vi "set_controls_enabled_state.vi"(8 "error in (no error)":errorcluster, 9 "status":T1(ring), 10 "control references":refnum<vi>[](array[refnum]), 11 "GenericPlugin in":refnum<class "GenericComponent.lvclass">) -> (0 "error out":errorcluster, 3 "GenericPlugin out":refnum<class "GenericComponent.lvclass">)   [LabVIEW 2010, in "GenericComponent.lvclass"]
uses:
  GenericComponent.lvclass
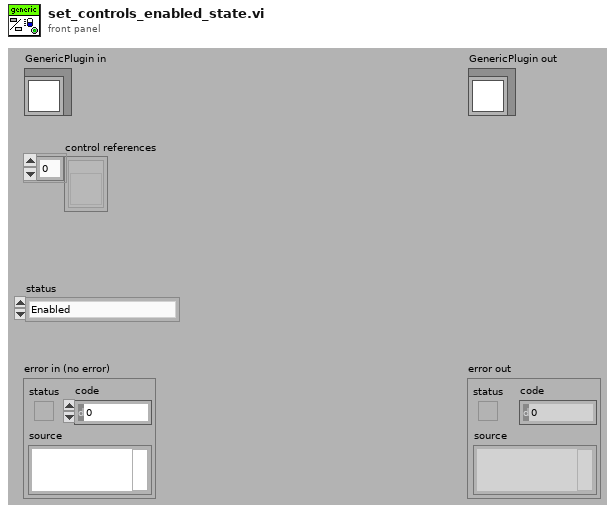
[diagram p1: front panel]
types:
  T1 = enum8{"Enabled", "Disabled", "Disabled and Grayed Out"}
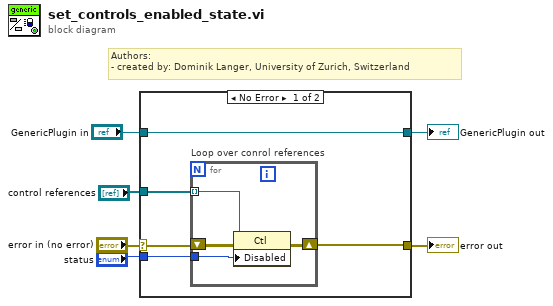
[diagram p0: block diagram]
diagram:
  # "Authors: \n- created by: Dominik Langer, University of Zurich, Switzerland"
  n1 = case shown="No Error" "error in (no error)" {
    selector: "error in (no error)" -> [w10 w17]
    tunnel: [w7 w17] -> w5
    tunnel: [w11 w16] -> w3
    tunnel: "GenericPlugin in" -> [w11 w16]
    tunnel: "control references" -> [w9 _]
    tunnel: "status" -> [w8 _]
    frame No Error {
      n2 = for "Loop over conrol references" {
        tunnel: w9 -> [w13] mode=indexing
        shift-right: [w14] -> w7
        shift-left: w10 -> [w15]
        tunnel: w8 -> [w12]
        n3 = property class="Ctl"(reference=w13, error in=w15, "Disabled"=w12) -> (error out=w14:errorcluster)  [unwired: 1 out]
      }
    }
    frame Error {
    }
  }
  "error out" <- w5
  "GenericPlugin out" <- w3
